vi "LMS on New GIC C.vi"(8 "Iteration num":dbl, 11 "GIC Input":T1={"     Use ?\nOff       On"=[FALSE, TRUE, FALSE, TRUE], "Mode:"=FALSE, "Extra Port"="", "Hokuyo Port"="COM7", "Tx Prop  Port"="COM6", "Compass Port"="", "GPS Port"="", "Num of WPs"=0, "WP Lats and Longs"={"WP Lats"=[], "WP Longs"=[]}, "Obst Lats and Longs"={"Obst Lats"=[], "Obst Longs"=[]}, "Parameters"=[], "GPS Data"=[], "Compass"=0.0, "LMS Vector"=[], "Vision Vector"=[], "Direction Cmd"=0.0, "Speed Cmd"=0.0, "WP Vector"=[], "WP Number"=0, "Extra"=0, "SW Map"=[], "Path Cluster"={"Path x node"=[], "Path y node"=[]}, "Sim Course"=[]} {"Obst Lats and Longs"."Obst Longs" format="%#_8g"; "Obst Lats and Longs"."Obst Lats" format="%#_8g"}) -> (3 "GIC Output":T1={"     Use ?\nOff       On"=[FALSE, TRUE, FALSE, TRUE], "Mode:"=FALSE, "Extra Port"="", "Hokuyo Port"="COM7", "Tx Prop  Port"="COM6", "Compass Port"="", "GPS Port"="", "Num of WPs"=0, "WP Lats and Longs"={"WP Lats"=[], "WP Longs"=[]}, "Obst Lats and Longs"={"Obst Lats"=[], "Obst Longs"=[]}, "Parameters"=[], "GPS Data"=[], "Compass"=0.0, "LMS Vector"=[], "Vision Vector"=[], "Direction Cmd"=0.0, "Speed Cmd"=0.0, "WP Vector"=[], "WP Number"=0, "Extra"=0, "SW Map"=[], "Path Cluster"={"Path x node"=[], "Path y node"=[]}, "Sim Course"=[]} {"Obst Lats and Longs"."Obst Longs" format="%#_8g"; "Obst Lats and Longs"."Obst Lats" format="%#_8g"})   [LabVIEW 2014]
uses:
  Hokuyo URG Series.lvlib
panel:
  in  "End Point":dbl=135.0
  in  "Start Point":dbl=-135.0
  in  "Cluster Count":dbl=1.0
  in  "Encoding Width":u16(ring)=3 items=["2 Byte"=2, "3 Byte"=3]
  in  "Scan Interval":dbl
  in  "Number of Scans":dbl
  out "Magnitude":dbl[](array[numeric])
  out "swmap":dbl[][](array[numeric])
  out "lms vector":dbl[](array[numeric])
  # "LMS on New GIC C"
  # "Input:"
  # "Output:"
  # "Iteration input:"
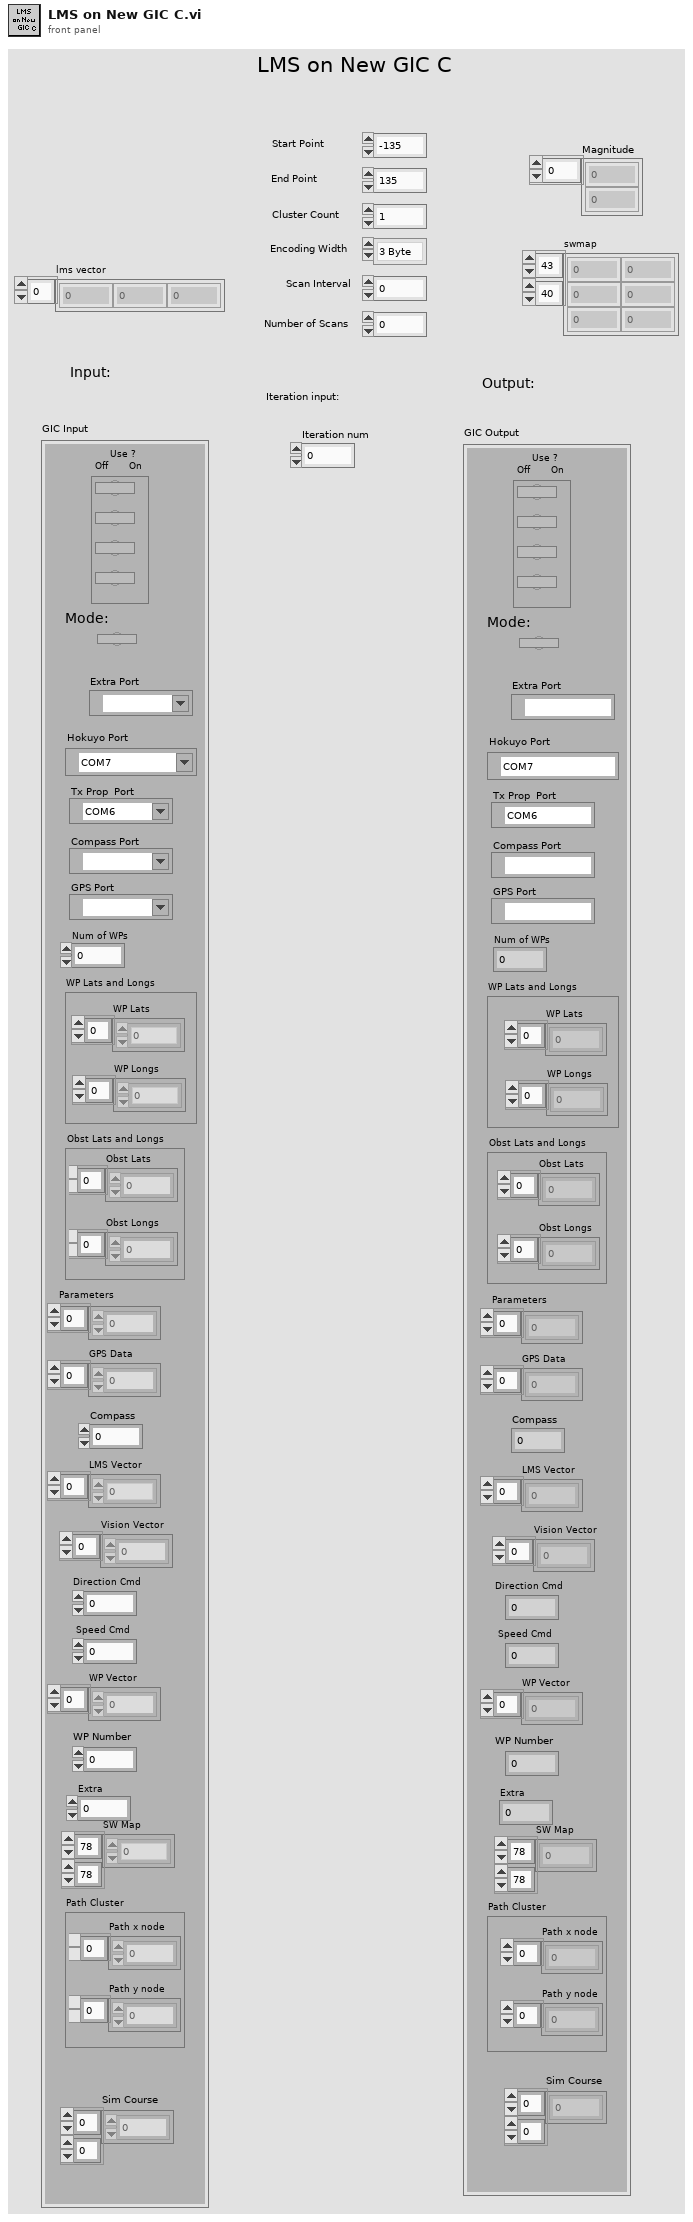
[diagram p1: front panel]
types:
  T1 = cluster{"     Use ?\nOff       On":bool[], "Mode:":bool, "Extra Port":refnum<visa-resource-name>, "Hokuyo Port":refnum<visa-resource-name>, "Tx Prop  Port":refnum<visa-resource-name>, "Compass Port":refnum<visa-resource-name>, "GPS Port":refnum<visa-resource-name>, "Num of WPs":i16, "WP Lats and Longs":cluster{"WP Lats":dbl[], "WP Longs":dbl[]}, "Obst Lats and Longs":cluster{"Obst Lats":dbl[], "Obst Longs":dbl[]}, "Parameters":dbl[], "GPS Data":dbl[], "Compass":dbl, "LMS Vector":dbl[], "Vision Vector":dbl[], "Direction Cmd":dbl, "Speed Cmd":dbl, "WP Vector":dbl[], "WP Number":i32, "Extra":i16, "SW Map":i32[][], "Path Cluster":cluster{"Path x node":dbl[], "Path y node":dbl[]}, "Sim Course":i8[][]}
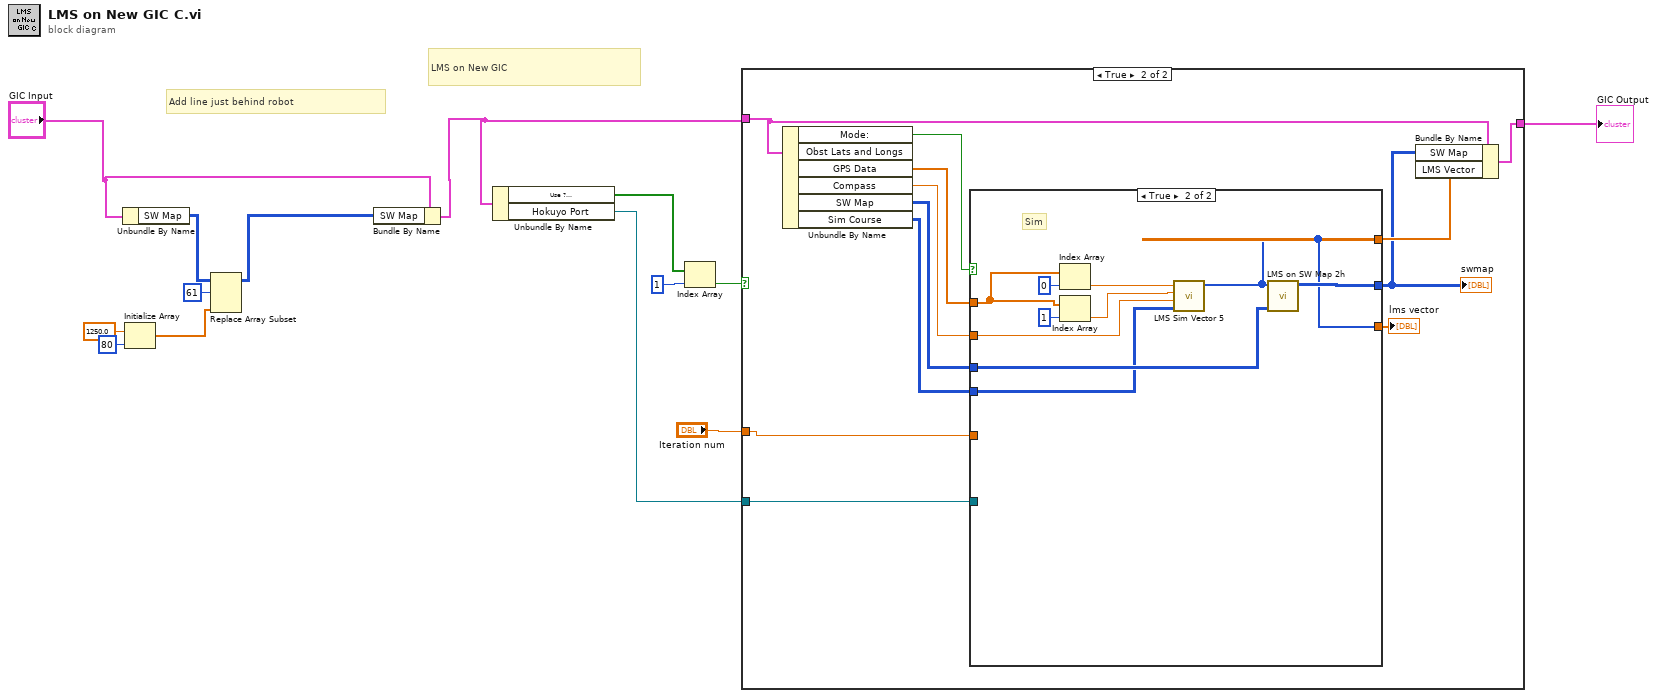
[diagram p0: block diagram]
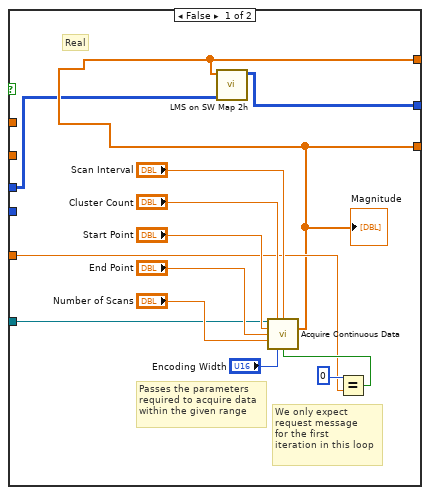
[diagram p3: hidden frame]
diagram:
  # "LMS on New GIC"
  # "Add line just behind robot"
  n1 = Unbundle By Name("GIC Input") -> ("SW Map"=w6:i32[][])
  n2 = Initialize Array(1250.0 ("element"), 80 ("dimension size")) -> (w4:dbl[])
  n3 = Replace Array Subset(array=w6, new element=w4, index (row)=61) -> (w3:i32[][])  [unwired: 1 in]
  n4 = Bundle By Name(cluster="GIC Input", "SW Map"=w3) -> (w1:T1)
  n5 = Unbundle By Name(w1) -> ("Use ?\nOff       On"=w14:bool[], "Hokuyo Port"=w9:refnum<visa-resource-name>)
  n6 = Index Array(array=w14, index=1) -> (element=w10:bool)
  n7 = case shown="True" w10 {
    tunnel: w1 -> [w15 w23]
    tunnel: [w15 w20] -> w12
    tunnel: w9 -> [_ w19]
    tunnel: "Iteration num" -> [_ w17]
    frame False {
    }
    frame True {
      n8 = Unbundle By Name(w23) -> ("Mode:"=w27:bool, "GPS Data"=w26:dbl[], "Compass"=w25:dbl, "SW Map"=w22:i32[][], "Sim Course"=w16:i8[][])  [unwired: 1 out]
      n9 = case shown="True" w27 {
        tunnel: w26 -> [_ w45]
        tunnel: w25 -> [_ w42]
        tunnel: w22 -> [w29 w50]
        tunnel: [w28 w49] -> w18
        tunnel: [w30 w48] -> w24
        tunnel: [w30 w48] -> w21
        tunnel: w19 -> [w34 _]
        tunnel: w17 -> [w31 _]
        tunnel: w16 -> [_ w41]
        frame False {
          # "We only expect\nrequest message\nfor the first\niteration in this loop"
          # "Passes the parameters\nrequired to acquire data\nwithin the given range"
          # "Real"
          n10 = Equal?(x=0, y=w31) -> (x = y?=w32:bool)
          n11 = call "Acquire Continuous Data.vi"("VISA resource name"=w34, "Cluster Count (1)"="Cluster Count", "Scan Interval (1)"="Scan Interval", "Start Point (-120°)"="Start Point", "End Point (120°)"="End Point", "Number of Scans (0)"="Number of Scans", "Data Encoding Width (3 Byte)"="Encoding Width", "Enable Request Message (F:Disable)"=w32) -> ("Magnitude"=w30:dbl[])  [unwired: 2 in, 5 out]
          "Magnitude" <- w30
          n12 = call "LMS on SW Map 2h.vi"("SW Map In"=w29, "LMS Vector"=w30) -> ("SW Map Out"=w28:i32[][])  [unwired: 9 in]
        }
        frame True {
          # "Sim"
          n13 = Index Array(array=w45, index=0) -> (element=w47:dbl)
          n14 = Index Array(array=w45, index=1) -> (element=w43:dbl)
          n15 = call "LMS Sim Vector 5.vi"("Sim Course"=w41, "Robot Heading"=w42, "Robot Long"=w43, "Robot Lat"=w47) -> ("dist"=w48:i32[])  [unwired: 7 in]
          n16 = call "LMS on SW Map 2h.vi"("SW Map In"=w50, "LMS Vector"=w48) -> ("SW Map Out"=w49:i32[][])  [unwired: 9 in]
        }
      }
      "lms vector" <- w21
      "swmap" <- w18
      n17 = Bundle By Name(cluster=w23, "SW Map"=w18, "LMS Vector"=w24) -> (w20:T1)
    }
  }
  "GIC Output" <- w12
